vi "SaveConfig.vi"(8 "error in (no error)":errorcluster, 11 "GRMActor in":refnum<class "StageController.lvclass">) -> (0 "error out":errorcluster, 3 "GRMActor out":refnum<class "StageController.lvclass">)   [LabVIEW 2020, in "StageController.lvlib" / "StageController.lvclass"]
uses:
  StageController.lvclass
  StageController.lvclass/StageController.ctl
  Model/Hardware Abstraction Layer/Component/GenericActor/GenericActor/GenericController.lvclass
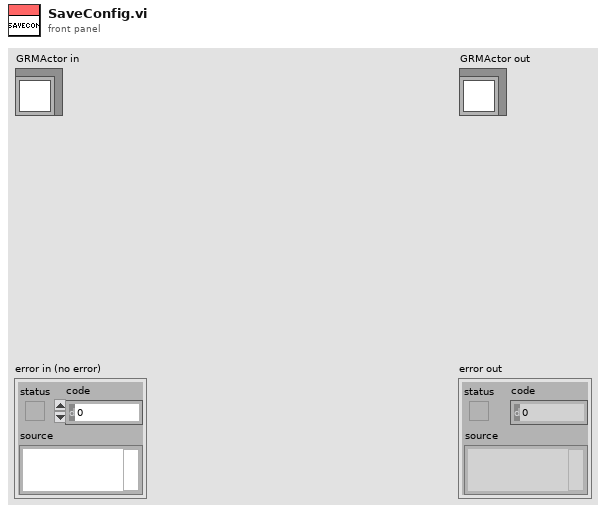
[diagram p1: front panel]
types:
  T1 = typedef "NI_LVConfig.lvlib/Config Data RefNum.ctl" = refnum<k1>
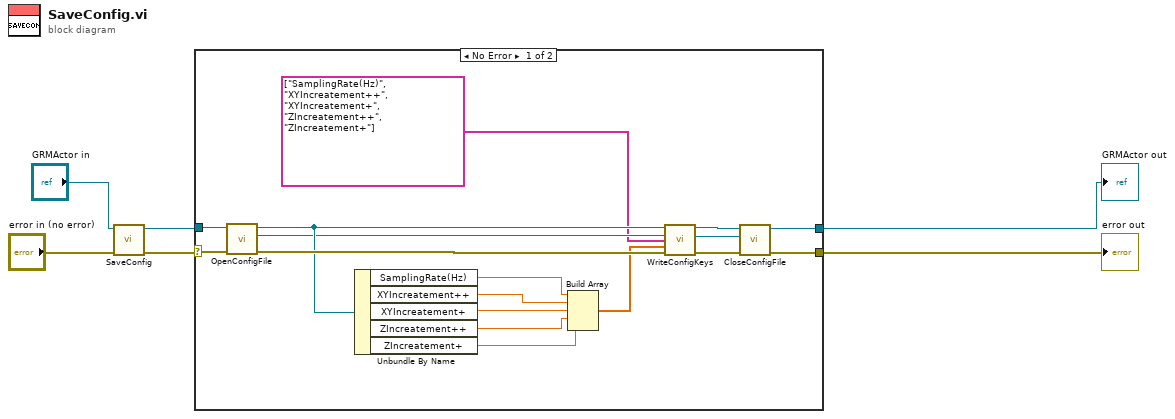
[diagram p0: block diagram]
diagram:
  n1 = call-parent "SaveConfig.vi"("error in (no error)"="error in (no error)", "GRMActor in"="GRMActor in") -> ("error out"=w3:errorcluster, "GRMActor out"=w4:refnum<class "StageController.lvclass">)  [unwired: 8 in]
  n2 = case shown="No Error" w3 {
    selector: w3 -> [w23 w24]
    tunnel: [w20 w24] -> w1
    tunnel: [w18 w25] -> w2
    tunnel: w4 -> [w17 w25]
    frame No Error {
      n3 = call-dynamic "OpenConfigFile.vi"("error in (no error)"=w23, "GRMActor in"=w17) -> ("error out"=w21:errorcluster, "refnum"=w15:T1, "GRMActor out"=w16:refnum<class "StageController.lvclass">)  [unwired: 7 in]
      n4 = Unbundle By Name(w16) -> ("SamplingRate(Hz)"=w12:dbl, "XYIncreatement++"=w11:dbl, "XYIncreatement+"=w10:dbl, "ZIncreatement++"=w9:dbl, "ZIncreatement+"=w8:dbl)
      n5 = Build Array(w12, w11, w10, w9, w8) -> (w7:dbl[])
      n6 = call-dynamic "WriteConfigKeys.vi"("GRMActor in"=w16, "Config Refnum"=w15, "Keys"=string[] ["SamplingRate(Hz)", "XYIncreatement++", "XYIncreatement+", "ZIncreatement++", "ZIncreatement+"] ("Values"), "DoubleValue"=w7, "error in (no error)"=w21) -> ("GRMActor out"=w19:refnum<class "StageController.lvclass">, "Config Refnum dup"=w14:T1, "error out"=w22:errorcluster)  [unwired: 8 in]
      n7 = call-dynamic "CloseConfigFile.vi"("error in (no error)"=w22, "refnum"=w14, "GRMActor in"=w19) -> ("error out"=w20:errorcluster, "GRMActor out"=w18:refnum<class "StageController.lvclass">)  [unwired: 7 in]
    }
    frame Error {
    }
  }
  "error out" <- w1
  "GRMActor out" <- w2
